vi "Math-Discrete Random Number.vi"(3 "replace?":bool, 4 "seed":i32=-1, 5 "N":i32=100, 6 "samples":i32=100) -> (1 "Random Values":i32[](array[numeric]))   [LabVIEW 2020]
uses:
  <vilib>/gmath/statdist.llb/Random Permutation.vi
  <vilib>/gmath/statdist.llb/Uniform (Discrete) Random.vi
  <vilib>/gmath/NI_Gmath.lvlib
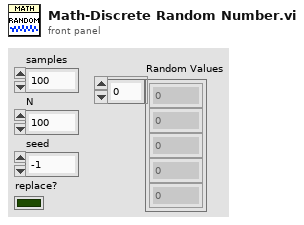
[diagram p1: front panel]
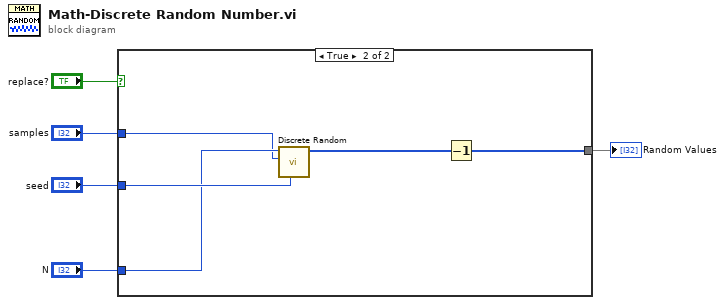
[diagram p0: block diagram]
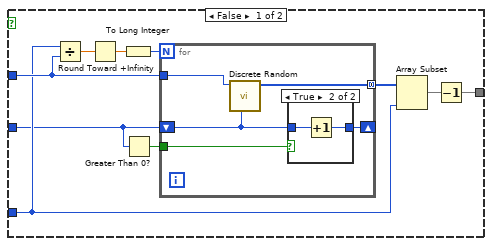
[diagram p2: hidden frame]
diagram:
  n1 = case shown="True" "replace?" {
    tunnel: "seed" -> [w7 w28]
    tunnel: "N" -> [w8 w25]
    tunnel: "samples" -> [w12 w24]
    tunnel: [w11 w26] -> w1
    frame False {
      n2 = Divide(x=w8, y=w12) -> (x/y=w15:dbl)
      n3 = Round Toward +Infinity(x=w15) -> (ceil(x): smallest int >= x=w14:dbl)
      n4 = To Long Integer(number=w14) -> (32bit integer=w13:i32)
      n5 = Greater Than 0?(x=w7) -> (x > 0?=w6:bool)
      n6 = for {
        N: w13 -> [_]
        shift-right: [w20] -> _
        shift-left: w7 -> [w19]
        tunnel: w12 -> [w18]
        tunnel: [w17] -> w10 mode=concatenating
        tunnel: w6 -> [w16]
        n7 = call-poly <vilib>:"Discrete Random.vi"("seed"=w19, "N"=w18) -> ("random permutation"=w17:i32[])  [unwired: 8 in, 1 out]
        n8 = case shown="True" w16 {
          tunnel: [w21 w23] -> w20
          tunnel: w19 -> [w21 w22]
          frame False {
          }
          frame True {
            n9 = Increment(x=w22) -> (x+1=w23:i32)
          }
        }
      }
      n10 = Array Subset(array=w10, length=w8) -> (w9:i32[])  [unwired: 1 in]
      n11 = Decrement(x=w9) -> (x-1=w11:i32[])
    }
    frame True {
      n12 = call-poly <vilib>:"Discrete Random.vi"("seed"=w28, "n"=w24, "samples"=w25) -> ("uniform (discrete) random data"=w27:i32[])  [unwired: 7 in, 1 out]
      n13 = Decrement(x=w27) -> (x-1=w26:i32[])
    }
  }
  "Random Values" <- w1
